vi "config_OSC.vi"() -> ()   [LabVIEW 2011]
uses:
  SubVIs/controls/scale.ctl
  SubVIs/controls/sampling_rate.ctl
  global.vi
  <instrlib>/Tektronix 7000 Series/Tektronix 7000 Series.lvlib
panel:
  in  "fastFrame mode":bool=TRUE caption="FastFrame"
  in  "fast frame count":i32
  in  "RESET?":bool
  in  "OSC":refnum<visa-resource-name>="OSC"
  in  "configure":bool
  out "resolution (Hz)":ext=24999.999999999999998 format="%#_6p"
  out "sampling interval (s)":ext=2e-10 format="%#_6p"
  out "waveform length (s)":ext=0.000040000000000000000003 format="%#_6p"
  in  "horizontal scale (t/div)":T1=0.0000040000000000000000001 items=["400ns/div", "1µs/div", "2µs/div", "4µs/div", "10µs/div", "20µs/div"]
  in  "sampling rate (Hz)":T2=5000000000.0 items=["20 GHz (50ps/sample)", "10 GHz (100ps/sample)", "5.0 GHz (200ps/sample)", "2.5 GHz (400ps/sample)", "1.25 GHz (0.8ns/sample)", "0.5 GHz (2ns/sample)"]
  out "sample points":i32=200000
  in  "Close":bool
  # "Configure Oscilloscope"
  # "Resolution and Record Length"
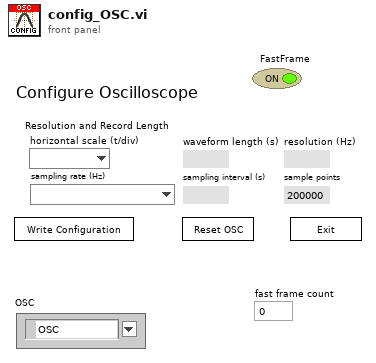
[diagram p1: front panel]
types:
  T1 = typedef "scale.ctl" = ext
  T2 = typedef "sampling_rate.ctl" = ext
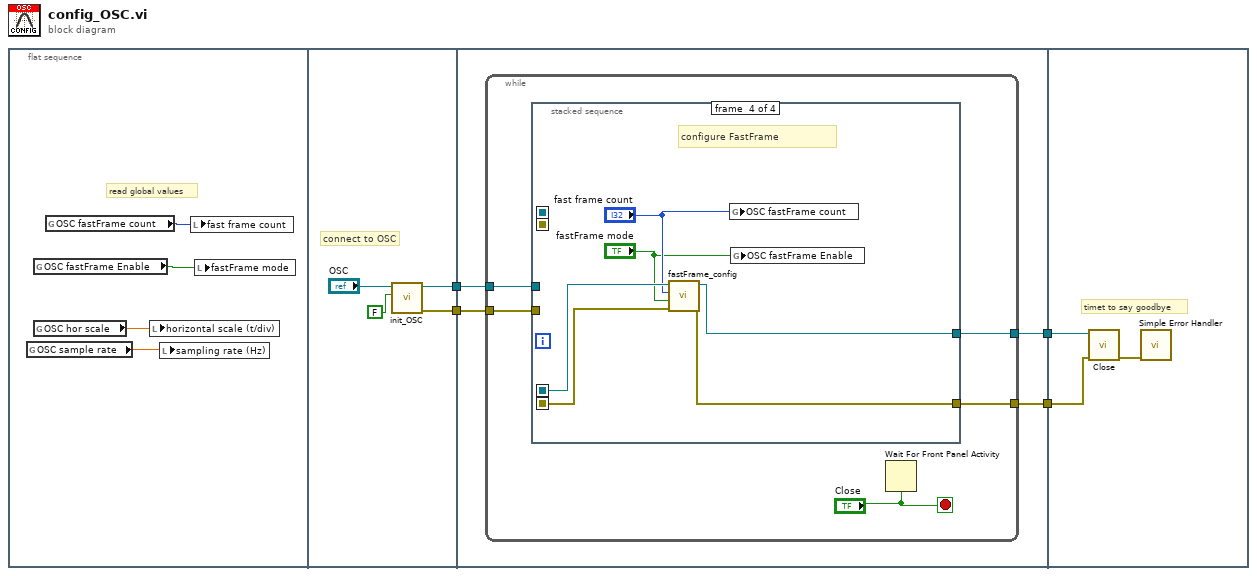
[diagram p0: block diagram]
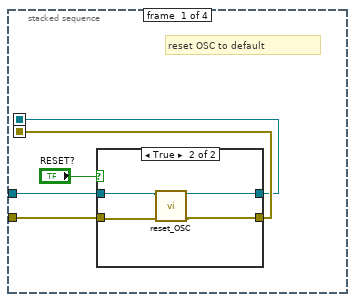
[diagram p2: hidden frame]
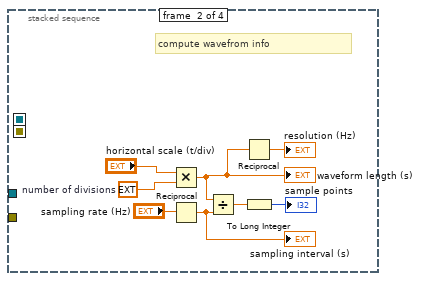
[diagram p4: hidden frame]
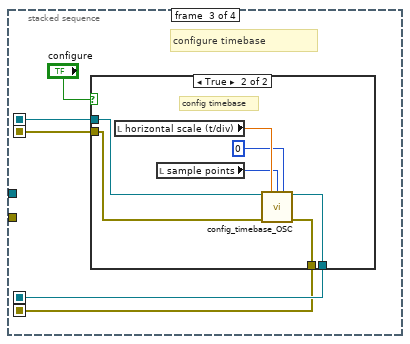
[diagram p5: hidden frame]
diagram:
  n1 = flat-sequence {
    tunnel: [w10] -> w4
    tunnel: [w9] -> w3
    tunnel: w4 -> [w15]
    tunnel: w3 -> [w16]
    tunnel: [w14] -> w2
    tunnel: [w13] -> w1
    tunnel: w2 -> [w62]
    tunnel: w1 -> [w61]
    frame #0 {
      # "read global values"
      n2 = global read "global.vi" "OSC sample rate"() -> (w7:T2)
      n3 = global read "global.vi" "OSC fastFrame Enable"() -> (w5:bool)
      n4 = global read "global.vi" "OSC hor scale"() -> (w8:T1)
      n5 = global read "global.vi" "OSC fastFrame count"() -> (w6:i32)
      n6 = local write "horizontal scale (t/div)"(w8) -> ()
      n7 = local write "sampling rate (Hz)"(w7) -> ()
      n8 = local write "fast frame count"(w6) -> ()
      n9 = local write "fastFrame mode"(w5) -> ()
    }
    frame #1 {
      # "connect to OSC"
      n10 = call "init_OSC.vi"("reset (f)"=FALSE, "VISA resource name"="OSC") -> ("error out"=w10:errorcluster, "VISA resource name out"=w9:refnum<visa-resource-name>)  [unwired: 8 in]
    }
    frame #2 {
      n11 = while {
        tunnel: w16 -> [w20]
        tunnel: w15 -> [w19]
        tunnel: [w18] -> w14
        tunnel: [w17] -> w13
        stop <- "Close" stop-if-true
        n12 = stacked-sequence {
          seq-local: [w22 _ _ _] -> [_ _ w42 _]
          seq-local: [w23 _ _ _] -> [_ _ w41 _]
          seq-local: [_ _ w44 _] -> [_ _ _ w60]
          seq-local: [_ _ w43 _] -> [_ _ _ w59]
          tunnel: w20 -> [w25 _ _ _]
          tunnel: w19 -> [w24 _ _ _]
          tunnel: [_ _ _ w58] -> w18
          tunnel: [_ _ _ w57] -> w17
          frame #0 {
            # "reset OSC to default"
            n13 = case shown="True" "RESET?" {
              tunnel: w25 -> [w27 w29]
              tunnel: w24 -> [w28 w30]
              tunnel: [w28 w31] -> w23
              tunnel: [w27 w32] -> w22
              frame False {
              }
              frame True {
                n14 = call "reset_OSC.vi"("error in (no error)"=w30, "VISA resource name"=w29) -> ("error out"=w31:errorcluster, "VISA resource name out"=w32:refnum<visa-resource-name>)  [unwired: 8 in]
              }
            }
          }
          frame #1 {
            w40 = ext 10.0  # number of divisions
            # "compute wavefrom info"
            n15 = Multiply(x="horizontal scale (t/div)", y=w40) -> (x*y=w34:T1)
            "waveform length (s)" <- w34
            n16 = Reciprocal(x="sampling rate (Hz)") -> (1/x=w37:T2)
            "sampling interval (s)" <- w37
            n17 = Divide(x=w34, y=w37) -> (x/y=w36:T1)
            n18 = Reciprocal(x=w34) -> (1/x=→"resolution (Hz)":T1)
            n19 = To Long Integer(number=w36) -> (32bit integer=→"sample points":i32)
          }
          frame #2 {
            # "configure timebase"
            n20 = case shown="True" "configure" {
              tunnel: [w47 w54] -> w44
              tunnel: w42 -> [w47 w48]
              tunnel: w41 -> [w46 w50]
              tunnel: [w46 w49] -> w43
              frame False {
              }
              frame True {
                # "config timebase"
                n21 = local read "horizontal scale (t/div)"() -> (w53:T1)
                n22 = local read "sample points"() -> (w51:i32)
                n23 = call "config_timebase_OSC.vi"("VISA resource name"=w48, "hor scale"=w53, "resolution"=w51, "Position"=0, "error in (no error)"=w50) -> ("VISA resource name out"=w54:refnum<visa-resource-name>, "error out"=w49:errorcluster)  [unwired: 9 in]
              }
            }
          }
          frame #3 {
            # "configure FastFrame"
            n24 = call "fastFrame_config.vi"("error in (no error)"=w59, "Fast Frame"="fastFrame mode", "fast frame count"="fast frame count", "VISA resource name"=w60) -> ("error out"=w57:errorcluster, "VISA resource name out"=w58:refnum<visa-resource-name>)  [unwired: 6 in]
            n25 = global write "global.vi" "OSC fastFrame count"("fast frame count") -> ()
            n26 = global write "global.vi" "OSC fastFrame Enable"("fastFrame mode") -> ()
          }
        }
        n27 = Wait For Front Panel Activity(3:"Close") -> ()  [unwired: 2 in, 1 out]
      }
    }
    frame #3 {
      # "timet to say goodbye"
      n28 = call <instrlib>:"Close.vi"("error in (no error)"=w61, "VISA resource name"=w62) -> ("error out"=w63:errorcluster)  [unwired: 9 in]
      n29 = call <vilib>:"Simple Error Handler.vi"("error in (no error)"=w63) -> ()  [unwired: 4 in, 5 out]
    }
  }
